vi "addDeviceListBox.vi"(8 "error in (no error)":errorcluster, 10 "new dev":string, 11 "reference":refnum<vi>) -> (0 "error out":errorcluster, 3 "reference out":refnum<vi>)   [LabVIEW 2010]
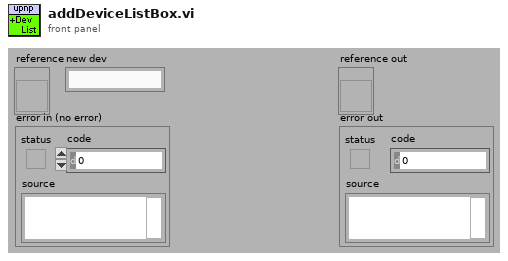
[diagram p1: front panel]
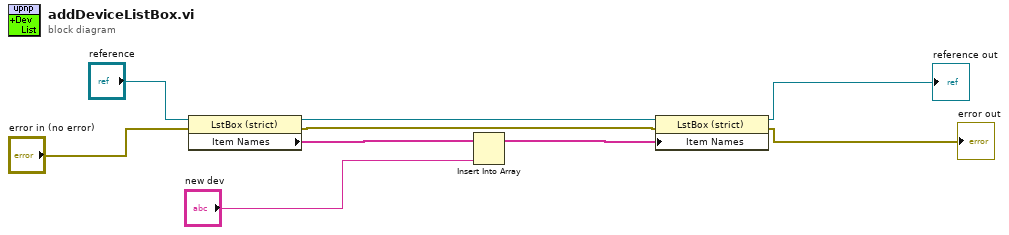
[diagram p0: block diagram]
diagram:
  n1 = property class="LstBox (strict)"(reference="reference", error in="error in (no error)") -> (reference out=w3:refnum<vi>, error out=w4:errorcluster, "Item Names"=w7:string[])
  n2 = Insert Into Array(array=w7, new element="new dev") -> (w6:string[])  [unwired: 1 in]
  n3 = property class="LstBox (strict)"(reference=w3, error in=w4, "Item Names"=w6) -> (reference out=→"reference out":refnum<vi>, error out=→"error out":errorcluster)
